vi "Entry.vi"(8 "error in (no error)":errorcluster, 10 "Context in":refnum<data-value>, 11 "Active in":refnum<class "Active.lvclass">) -> (0 "error out":errorcluster, 2 "Context out":refnum<data-value>, 3 "Active out":refnum<class "Active.lvclass">)   [LabVIEW 2024, in "State.lvlib" / "Active.lvclass"]
uses:
  Active.lvclass
  Context/Context/Context.lvclass
  <vilib>/ActorFramework/Message Enqueuer/Message Enqueuer.lvclass/Message Enqueuer.ctl
  <vilib>/ActorFramework/Message Enqueuer/Enqueue.vi
  State Machine Messages/Start Logging Msg/Start Logging Msg.lvclass
  C:/Program Files (x86)/National Instruments/LabVIEW 2024/vi.lib/ActorFramework/Message/Message.lvclass
  <vilib>/ActorFramework/Message Priority Queue/Priority Enqueue.vi
  <vilib>/ActorFramework/Message Enqueuer/Message Enqueuer.lvclass
  Active.lvclass/Active.ctl
panel:
  # "ENTRY!"
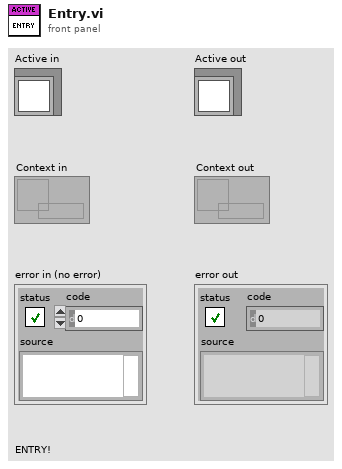
[diagram p1: front panel]
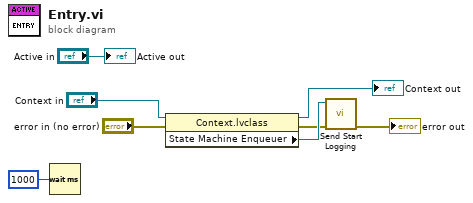
[diagram p0: block diagram]
diagram:
  n1 = Wait (ms)(milliseconds to wait=u32 1000) -> ()  [unwired: 1 out]
  n2 = property class="Context.lvclass"(reference="Context in", error in="error in (no error)") -> (reference out=→"Context out":refnum<data-value>, error out=w1:errorcluster, "State Machine Enqueuer"=w2:refnum<class "Message Enqueuer.lvclass">)
  n3 = call "Send Start Logging.vi"("error in (no error)"=w1, "Message Enqueuer"=w2) -> ("error out"=→"error out":errorcluster)  [unwired: 8 in, 1 out]
  "Active out" <- "Active in"
